vi "Dispose.vi"(8 "error in (no error)":errorcluster, 11 "JsonEvents in":refnum<class "JsonEvents.lvclass">) -> (0 "error out":errorcluster, 3 "JsonEvents out":refnum<class "JsonEvents.lvclass">)   [LabVIEW 2020, in "wamplv.lvlib" / "JsonEvents.lvclass"]
uses:
  JsonEvents.lvclass
  JsonEvents.lvclass/JsonEvents.ctl
  EventsParent/Events.lvclass
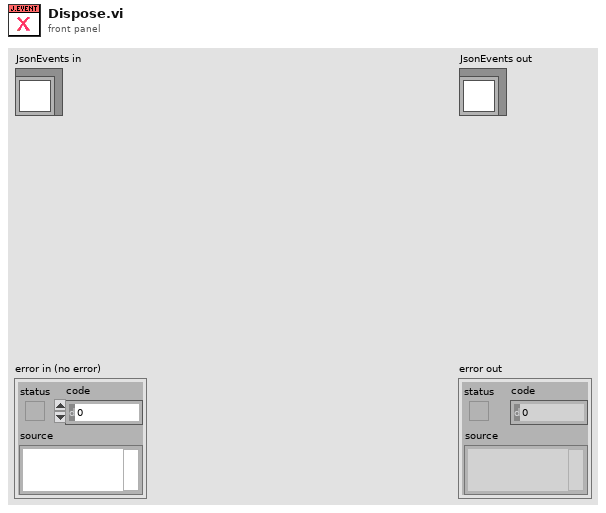
[diagram p1: front panel]
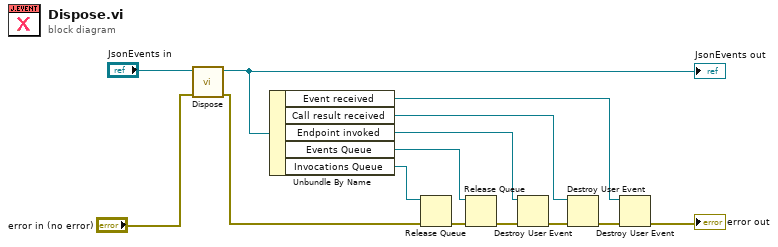
[diagram p0: block diagram]
diagram:
  n1 = call-parent "Dispose.vi"("error in (no error)"="error in (no error)", "EventsParent in"="JsonEvents in") -> ("error out"=w1:errorcluster, "EventsParent out"=w6:refnum<class "JsonEvents.lvclass">)  [unwired: 8 in]
  "JsonEvents out" <- w6
  n2 = Unbundle By Name(w6) -> ("Event received"=w8:refnum<user-event>, "Call result received"=w10:refnum<user-event>, "Endpoint invoked"=w12:refnum<user-event>, "Events Queue"=w4:refnum<queue>, "Invocations Queue"=w2:refnum<queue>)
  n3 = Release Queue(queue=w2, error in (no error)=w1) -> (error out=w3:errorcluster)  [unwired: 1 in, 2 out]
  n4 = Release Queue(queue=w4, error in (no error)=w3) -> (error out=w5:errorcluster)  [unwired: 1 in, 2 out]
  n5 = Destroy User Event(user event=w12, error in=w5) -> (error out=w11:errorcluster)
  n6 = Destroy User Event(user event=w10, error in=w11) -> (error out=w9:errorcluster)
  n7 = Destroy User Event(user event=w8, error in=w9) -> (error out=→"error out":errorcluster)
